vi "Numeric.vi"(8 "error in":errorcluster, 11 "GObj Refnum":refnum<vi>) -> (0 "error out":errorcluster, 3 "Numeric out":refnum<class "Numeric.lvclass">)   [LabVIEW 2014, in "Numeric.lvclass"]
uses:
  Numeric.lvclass
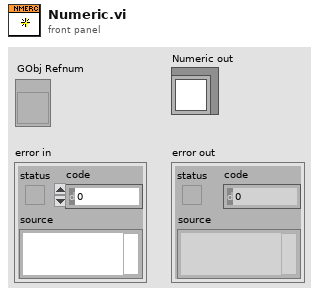
[diagram p1: front panel]
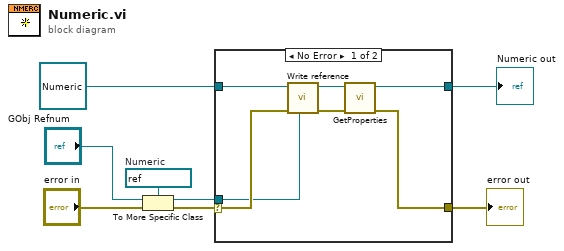
[diagram p0: block diagram]
diagram:
  w3 = refnum<vi> refnum  # Numeric
  n1 = To More Specific Class(target class=w3, reference="GObj Refnum", error in="error in") -> (specific class reference=w1:refnum<vi>, error out=w2:errorcluster)
  n2 = case shown="No Error" w2 {
    selector: w2 -> [w14 w17]
    tunnel: [w9 w17] -> w8
    tunnel: [w10 w16] -> w6
    tunnel: refnum<class "Numeric.lvclass"> refnum ("Decoration in") -> [w15 w16]
    tunnel: w1 -> [w13 _]
    frame No Error {
      n3 = call-dynamic "Write reference.vi"("reference"=w13, "error in"=w14, "GObject in"=w15) -> ("error out"=w11:errorcluster, "GObject out"=w12:refnum<class "Numeric.lvclass">)  [unwired: 5 in]
      n4 = call-dynamic "GetProperties.vi"("error in"=w11, "Numeric in"=w12) -> ("error out"=w9:errorcluster, "Numeric out"=w10:refnum<class "Numeric.lvclass">)  [unwired: 8 in]
    }
    frame Error {
    }
  }
  "error out" <- w8
  "Numeric out" <- w6
